vi "_check controller.vi"() -> ()   [LabVIEW 2017]
uses:
  <vilib>/Simulation/Scripting/Companion Diagram/SimConfigNode/SimParams.ctl
  <vilib>/Simulation/Scripting/Companion Diagram/SimConfigNode/_simSolvers.ctl
  <vilib>/Simulation/Implementation/Shared/SIMSCR Execution Mode.ctl
  <vilib>/Simulation/Param Hierarchy/Typedefs/SIMPH Param Control Actions.ctl
  <vilib>/Simulation/Implementation/Shared/NILVSim_ParamChanged.vi
  <vilib>/Simulation/Implementation/Shared/NILVSIM_BeginStep.vi
  <vilib>/Simulation/Implementation/Shared/NILVSim_Manager.vi
  <vilib>/Utility/error.llb/Clear Errors.vi
  <vilib>/Simulation/Implementation/Shared/NILVSim_FinalizeModel.vi
  <vilib>/DAQmx/read.llb/DAQmx Read (Counter DBL 1Chan 1Samp).vi
  <vilib>/DAQmx/read.llb/DAQmx Read (Digital Bool 1Line 1Point).vi
  917b7e52-755f-4d44-bea8-9e7c9beac24e.vi
  a58f9967-76f1-4ebc-ad3d-26e75a3ca160.vi
  <vilib>/DAQmx/write.llb/DAQmx Write (Analog DBL 1Chan 1Samp).vi
  <vilib>/DAQmx/create/channels.llb/DAQmx Create Channel (AO-Voltage-Basic).vi
  <vilib>/DAQmx/create/channels.llb/DAQmx Create Channel (DI-Digital Input).vi
  <vilib>/DAQmx/create/channels.llb/DAQmx Create Channel (CI-Count Edges).vi
  <vilib>/Simulation/Implementation/Shared/SIM Unbundle Sim Info.vi
  <vilib>/Simulation/Implementation/Shared/NILVSim_Initialize.vi
  <vilib>/Simulation/Utility/Implementation/NILVSim Get Time and IsAcceptedStep.vi
  <vilib>/Simulation/Implementation/Shared/SIMSH Read Queue.vi
  <vilib>/Simulation/Implementation/Shared/NILVSim_GetModelError.vi
  <vilib>/Simulation/Implementation/Shared/SIM Bundle Sim Info.vi
  <vilib>/DAQmx/miscellaneous.llb/DAQmx Fill In Error Info.vi
  <vilib>/Simulation/Implementation/XNodeFramework/SimXNode/SimX.xnode
  <vilib>/Simulation/Model Libraries/PID/SIM PID (Parallel).vi
  <vilib>/Simulation/Model Libraries/PID/SIM PID.vi
  <vilib>/Simulation/Scripting/Companion Diagram/SimConfigNode/SimDog.xnode
  <vilib>/Simulation/Model Libraries/PID/SIM PID (Academic).vi
  <vilib>/Simulation/Implementation/Shared/NI_SIM_Implementation.lvlib
panel:
  out "temp height":dbl
  out "Boolean 2":bool
  out "reset":bool
  in  "checking re":bool
  in  "checking enums":T1(ring)
  in  "rectangle":bool
  in  "Boolean":bool
  out "prev index":dbl
  out "Point rectangle is drawing":dbl
  out "Rectangle Y":dbl[](array[numeric])
  out "Rectangle X":dbl[](array[numeric])
  in  "stage rectangle":T2(ring)
  out "Step 2I":bool
  out "Step 2G":bool
  out "Step 2E":bool
  out "stay1":dbl
  out "stay":dbl
  out "calculating error x":dbl
  out "calculating error y":dbl
  in  "origin":bool
  out "Previous Y":dbl
  out "Previous X":dbl
  out "Current Y":dbl
  out "Current X":dbl
  out "previous index":dbl
  out "both/reset enter":bool
  out "reset complete":bool
  out "x circle":bool
  out "y circle":bool
  out "Point circle is drawing":dbl
  out "false":bool
  in  "Radius 2":dbl
  out "No of Points":dbl
  out "Passing Y":dbl
  out "Y array":dbl[](array[numeric])
  out "array Y length 2":dbl
  out "Passing X":dbl
  out "X array":dbl[](array[numeric])
  out "array x Length 2":dbl
  in  "stage circle":T2(ring)
  in  "check instruc":bool
  out "x entered":dbl
  out "y enetred":dbl
  out "greater -1 x":bool
  out "less 1 x":bool
  out "direction selected":dbl
  out "at 2f":bool
  out "Step 2J":bool
  out "Step 2H":bool
  out "Shape drawing steps":enum16{"corner", "1st switch", "reverse"}(ring)
  out "Step 2D":bool
  out "c":bool
  in  "height":dbl
  in  "length":dbl
  in  "part":T3(ring)=enum."a"
  in  "Has encoders been reset?":enum16{"don't reset", "reset"}(ring)
  out "x distance currently being travelled":dbl
  out "y distance currently being travelled":dbl
  out "error calced":dbl
  out "p1 dis 2":dbl
  out "p1 dis":dbl
  out "error y":dbl
  out "calc distance y":dbl
  out "calc distanc x":dbl
  out "error x":dbl
  out "reached y":bool
  out "reached x":bool
  out "Numeric":dbl
  in  "Draw rectangle":bool
  in  "Draw circle":bool
  out "In drawing mode":bool
  in  "Right-Down":bool
  in  "Left-Up":bool
  in  "Left-Down":bool
  in  "Right-Up":bool
  in  "right":bool
  in  "left":bool
  in  "motor 2":dbl(slide)=1.5 scale=-10.0..10.0
  in  "down":bool
  in  "up":bool
  in  "Y Length":dbl=30.0
  in  "X Length":dbl=30.0
  in  "Motor 2 encoder":tag="Dev1/ctr1"
  out "Pulses M2":dbl format="%.2f"
  in  "Motor 1 encoder":tag="Dev1/ctr0"
  out "Pulses M1":dbl format="%.2f"
  out "Right":bool
  out "Bottom":bool
  out "Left":bool
  out "Top":bool
  in  "Switch 4/Line 3":tag="Dev1/port0/line3"
  in  "Switch 3/Line 2":tag="Dev1/port0/line2"
  in  "Switch 2/Line 1":tag="Dev1/port0/line1"
  in  "Switch 1/Line 0":tag="Dev1/port0/line0"
  in  "Motor stop":bool
  in  "Motor 1":tag="Dev1/ao0"
  in  "max Voltage":dbl=10.0
  in  "Min Voltage":dbl=-10.0
  in  "Motor 2":tag="Dev1/ao1"
  in  "motor 1":dbl(slide)=1.5 scale=-10.0..10.0
  in  "stop":bool
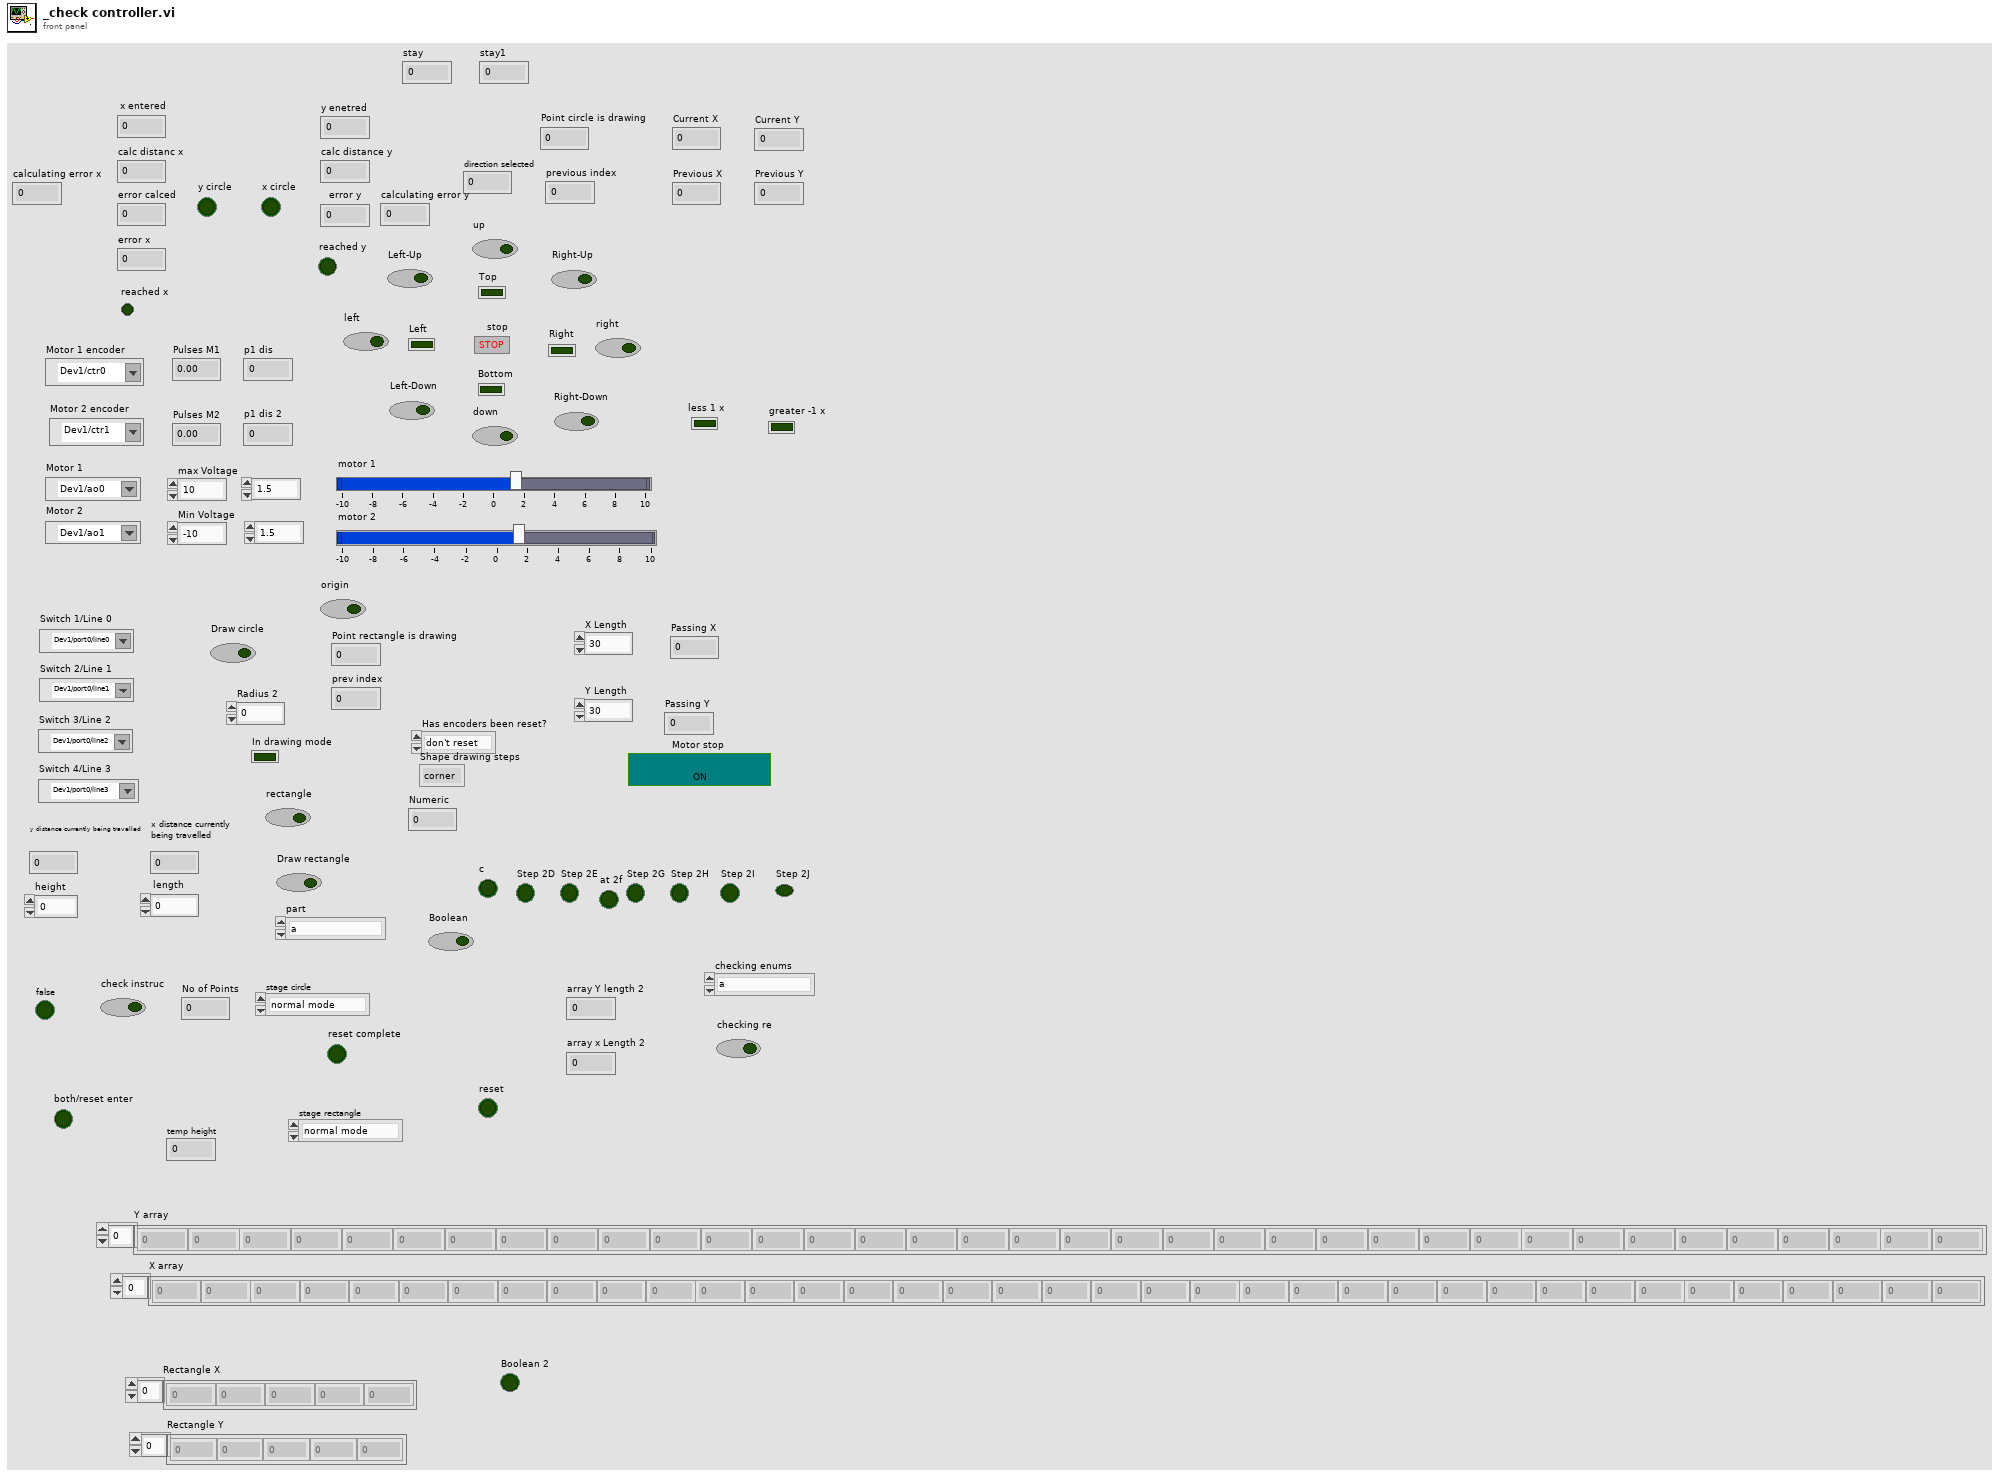
[diagram p1: front panel]
types:
  T1 = enum16{"a", "starting pt", "reset", "going right", "reset before down", "going down", "reset before left", "going left", "reset before up", "going up", "nothing"}
  T2 = enum16{"normal mode", "take to origin", "reset before start", "create points", "draw points", "checking if draw", "reset draw counter"}
  T3 = enum16{"nothing", "j", "i", "h", "g", "f", "e", "d", "c", "b", "a"}
  T4 = enum16{"a", "starting pt", "reset", "going right", "reset before down", "going down", "reset before left", "going left", "reset before up", "going up"}
  T5 = enum16{"Simulate to Completion", "Single Time-Step Simulation (Fixed Step Only)"}
  T6 = typedef "SIMSCR Execution Mode.ctl" = enum16{"Simulate to Completion", "Single Time-Step Simulation (Fixed Step Only)"}
  T7 = typedef "SIMPH Param Control Actions.ctl" = enum16{"get params", "set params"}
  T8 = cluster{"SIMSH Sim Time":dbl, "SIM PID Derivative Gain.vi":cluster{"output":dbl}, "SIM PID Derivative Gain.vi - SIMSH":cluster{"SIMSH Sim Time":dbl, "t 3":dbl, "Select 2":cluster{"s? t:f":dbl}, "Equal?":cluster{"x = y?":bool}, "Or":cluster{"x .or. y?":bool}, "Equal To 0?":cluster{"x = 0?":bool}}, "High Frequency [s] (Tf)":dbl, "Gain":cluster{"output":dbl}, "Summation":cluster{"Result":dbl}, "Integral Gain - series.vi":cluster{"output":dbl}, "Integral Gain - series.vi - SIMSH":cluster{"SIMSH Sim Time":dbl, "Select 2":cluster{"s? t:f":dbl}, "integral in gain?":bool, "Integrator":cluster{"output y(t)":dbl}, "Gain 2":cluster{"output":dbl}, "Select":cluster{"s? t:f":dbl}, "Equal To 0?":cluster{"x = 0?":bool}, "Reciprocal":cluster{"1/x":dbl}}}
  T9 = typedef "SimParams.ctl" = cluster{"Initial Time (s)":dbl, "Final Time (s)":dbl, "Step Size (s)":dbl, "ODE Solver":T10, "Minimum Step Size (s)":dbl, "Maximum Step Size (s)":dbl, "Relative Tolerance":dbl, "Absolute Tolerance":dbl, "Software Timing":bool, "Initial Step Size (s)":dbl, "Automatic Fixed Step Size?":bool, "Automatic Discrete Step Size?":bool, "Discrete Step Size (s)":dbl, "Calculate using Time Step":bool, "Solver Wired?":bool, "Prev.Frm.Expected End":u64, "Prev.Frm.Actual End":u64, "Prev.Frm.Finished Late?":bool, "Prev.Iter.Expected End":u64, "Prev.Iter.Actual End":u64, "Prev.Iter.Finished Late?":bool, "Expected Iteration Start":u64, "Actual Iteration Start":u64, "Expected Frame Start":u64, "Actual Frame Start":u64, "Source Name":string, "Name":string, "Period":i64, "Deadline":i64, "Offset":i64, "Start":i64, "Priority":i32, "Timeout":i32, "Processor":i32, "Mode":enum32{"No Change", "Process missed periods, maintain original phase", "Discard missed periods, maintain original phase", "Process missed periods, ignore original phase", "Discard missed periods, ignore original phase"}, "Wakeup reason":enum32{"Normal", "Aborted", "Asynchronous wakeup", "Timing source error", "Timed loop error", "Timeout"}, "Error":errorcluster, "Source Type":string, "Secondary Source Type":string, "Global End Time":u64, "Global Start Time":u64, "Full Solver Reset":bool, "Execution Mode":T6, "Nan/Inf Check":bool, "Custom Solver Library":string, "Solver Is Variable":bool, "custom solver name":string, "Signal Collection Decimation":u32}
  T10 = typedef "_simSolvers.ctl" = enum16{"Runge-Kutta 1 (Euler)", "Runge-Kutta 2", "Runge-Kutta 3", "Runge-Kutta 4", "Runge-Kutta 23 (variable)", "Runge-Kutta 45 (variable)", "BDF (variable)", "Adams-Moulton (variable)", "Rosenbrock (variable)", "Discrete States Only", "SDIRK 4 (variable)", "Radau 5 (variable)", "Radau 9 (variable)", "Radau 13 (variable)", "Radau [Variable Order] (variable)", "Gear's Method (variable)", "Linearizer", "State Query", "Trim Eval", "Custom Solver"}
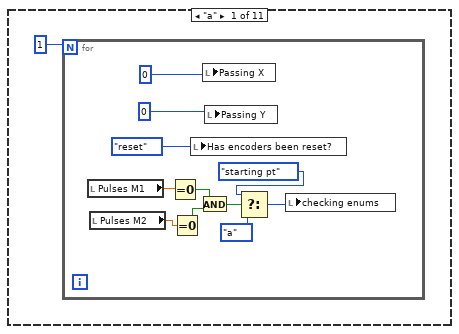
[diagram p3: hidden frame]
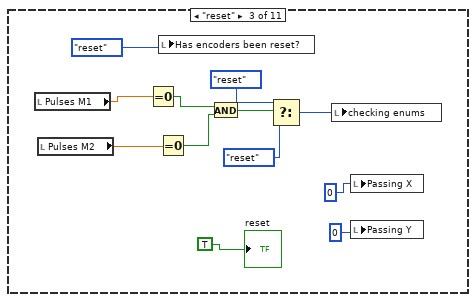
[diagram p4: hidden frame]
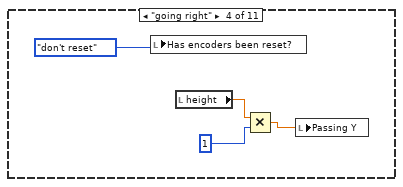
[diagram p5: hidden frame]
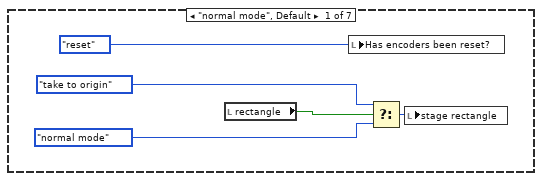
[diagram p14: hidden frame]
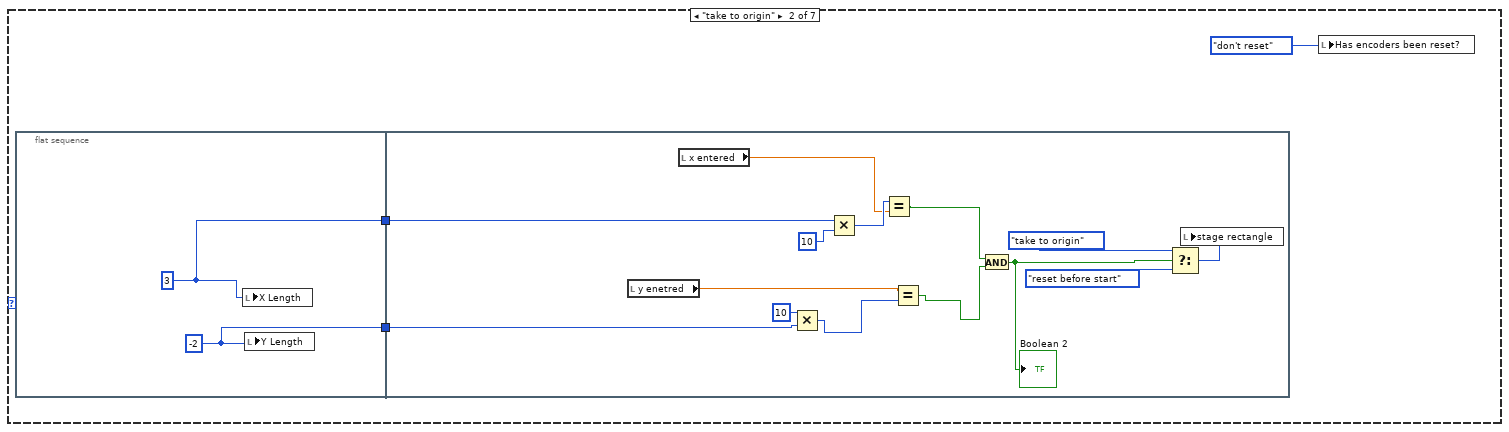
[diagram p15: hidden frame]
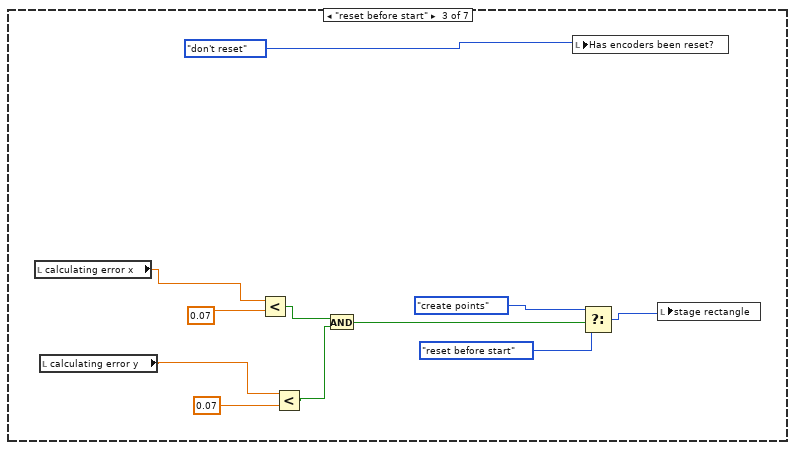
[diagram p16: hidden frame]
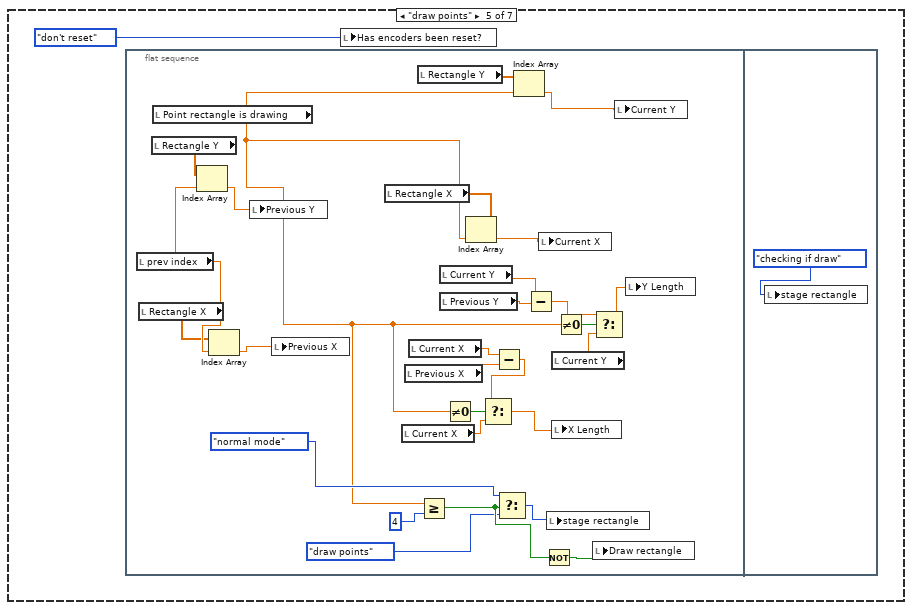
[diagram p17: hidden frame]
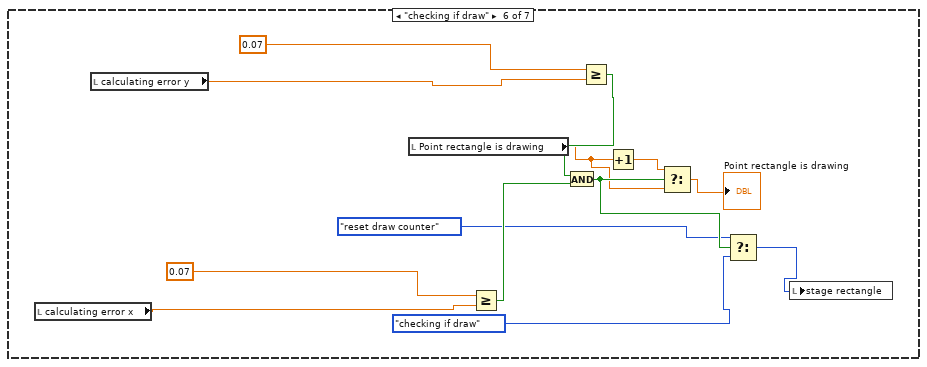
[diagram p18: hidden frame]
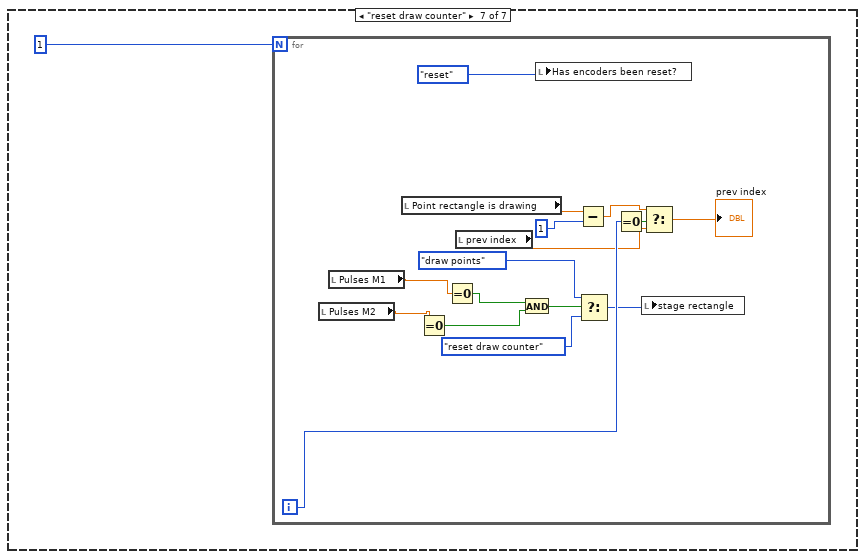
[diagram p19: hidden frame]
diagram:
  n1 = call-poly <vilib>:"DAQmx Create Virtual Channel.vi"("lines"="Switch 1/Line 0") -> ("task out"=w36:refnum<k21>, "error out"=w32:errorcluster)  [unwired: 13 in]
  n2 = call-poly <vilib>:"DAQmx Create Virtual Channel.vi"("lines"="Switch 2/Line 1") -> ("task out"=w35:refnum<k21>, "error out"=w31:errorcluster)  [unwired: 13 in]
  n3 = call-poly <vilib>:"DAQmx Create Virtual Channel.vi"("lines"="Switch 3/Line 2") -> ("task out"=w34:refnum<k21>, "error out"=w30:errorcluster)  [unwired: 13 in]
  n4 = call-poly <vilib>:"DAQmx Create Virtual Channel.vi"("lines"="Switch 4/Line 3") -> ("task out"=w33:refnum<k21>, "error out"=w29:errorcluster)  [unwired: 13 in]
  n5 = call-poly <vilib>:"DAQmx Create Virtual Channel.vi"("maximum value"="max Voltage", "minimum value"="Min Voltage", "physical channels"="Motor 1") -> ("task out"=w46:refnum<k21>, "error out"=w42:errorcluster)  [unwired: 11 in]
  n6 = call <vilib>:"DAQmx Start Task.vi"("task/channels in"=w36, "error in"=w32) -> ("task out"=w28:refnum<k21>, "error out"=w26:errorcluster)  [unwired: 12 in]
  n7 = call <vilib>:"DAQmx Start Task.vi"("task/channels in"=w35, "error in"=w31) -> ("task out"=w24:refnum<k21>, "error out"=w21:errorcluster)  [unwired: 12 in]
  n8 = call-poly <vilib>:"DAQmx Create Virtual Channel.vi"("maximum value"="max Voltage", "minimum value"="Min Voltage", "physical channels"="Motor 2") -> ("task out"=w49:refnum<k21>, "error out"=w41:errorcluster)  [unwired: 11 in]
  n9 = call-poly <vilib>:"DAQmx Create Virtual Channel.vi"("counter"="Motor 1 encoder") -> ("task out"=w7:refnum<k21>, "error out"=w2:errorcluster)  [unwired: 13 in]
  n10 = call-poly <vilib>:"DAQmx Create Virtual Channel.vi"("counter"="Motor 2 encoder") -> ("task out"=w6:refnum<k21>)  [unwired: 13 in, 1 out]
  n11 = call <vilib>:"DAQmx Start Task.vi"("task/channels in"=w34, "error in"=w30) -> ("task out"=w23:refnum<k21>, "error out"=w20:errorcluster)  [unwired: 12 in]
  n12 = call <vilib>:"DAQmx Start Task.vi"("task/channels in"=w33, "error in"=w29) -> ("task out"=w22:refnum<k21>, "error out"=w19:errorcluster)  [unwired: 12 in]
  n13 = call <vilib>:"DAQmx Start Task.vi"("task/channels in"=w7) -> ("task out"=w3:refnum<k21>)  [unwired: 13 in, 1 out]
  n14 = call <vilib>:"DAQmx Start Task.vi"("task/channels in"=w6) -> ("task out"=w1:refnum<k21>)  [unwired: 13 in, 1 out]
  n15 = while {
    tunnel: w49 -> [w242]
    tunnel: [w239] -> w48
    tunnel: w46 -> [w236]
    tunnel: [w235] -> w45
    tunnel: w42 -> [w233]
    tunnel: w41 -> [w232]
    tunnel: w28 -> [w226]
    tunnel: [w225] -> w27
    tunnel: w26 -> [w224]
    tunnel: [w223] -> w25
    tunnel: w24 -> [w222]
    tunnel: w23 -> [w221]
    tunnel: w22 -> [w220]
    tunnel: w21 -> [w219]
    tunnel: w20 -> [w218]
    tunnel: w19 -> [w217]
    tunnel: [w216] -> w18
    tunnel: [w215] -> w17
    tunnel: [w214] -> w16
    tunnel: [w213] -> w15
    tunnel: [w212] -> w14
    tunnel: [w211] -> w13
    tunnel: [w147] -> w10
    tunnel: w3 -> [w149]
    tunnel: w2 -> [w148]
    tunnel: w1 -> [w145]
    stop <- "stop" stop-if-true
    n16 = case shown="True" "check instruc" {
      frame False {
        "false" <- TRUE
      }
      frame True {
        n17 = case shown="\"checking if draw\"" "stage circle" {
          frame "normal mode", Default {
            n18 = local read "check instruc"() -> (w574:bool)
            n19 = local write "Y Length"(0) -> ()
            n20 = local write "X Length"(0) -> ()
            n21 = local write "Has encoders been reset?"(enum16{"don't reset", "reset"}."reset") -> ()
            n22 = Select(t=T2."create points", s=w574, f=T2."normal mode") -> (s? t:f=w575:T2)
            n23 = local write "stage circle"(w575) -> ()
          }
          frame "take to origin" {
            n24 = local write "stage circle"(T2."reset before start") -> ()
            n25 = local write "Has encoders been reset?"(enum16{"don't reset", "reset"}."don't reset") -> ()
          }
          frame "reset before start" {
            n26 = local read "Pulses M1"() -> (w589:dbl)
            n27 = local read "Pulses M2"() -> (w587:dbl)
            n28 = Equal?(x=w589, y=0) -> (x = y?=w584:bool)
            n29 = Equal?(x=w587, y=0) -> (x = y?=w585:bool)
            n30 = local write "Y Length"(0) -> ()
            n31 = local write "X Length"(0) -> ()
            n32 = And(x=w584, y=w585) -> (x .and. y?=w583:bool)
            n33 = local write "Has encoders been reset?"(enum16{"don't reset", "reset"}."reset") -> ()
            n34 = Select(t=T2."create points", s=w583, f=T2."reset before start") -> (s? t:f=w580:T2)
            n35 = local write "stage circle"(w580) -> ()
          }
          frame "create points" {
            n36 = for {
              N: 88 -> [_]
              shift-right: [w609] -> w600
              shift-left: _ -> [_]
              tunnel: [w609] -> w605 mode=indexing
              shift-right: [w608] -> w602
              shift-left: _ -> [_]
              tunnel: [w608] -> w604 mode=indexing
              i -> [w610]
              n37 = Multiply(x=2, y=3.141592653589793) -> (x*y=w613:dbl)
              n38 = Increment(x=w610) -> (x+1=w611:i32)
              n39 = Divide(x=w613, y=88) -> (x/y=w615:dbl)
              n40 = Multiply(x=w615, y=w611) -> (x*y=w612:dbl)
              n41 = Cosine(x=w612) -> (cos(x)=w618:dbl)
              n42 = Sine(x=w612) -> (sin(x)=w619:dbl)
              n43 = Multiply(x=w619, y="Radius 2") -> (x*y=w609:dbl)
              n44 = Multiply(x=w618, y="Radius 2") -> (x*y=w608:dbl)
              "No of Points" <- w610
            }
            "Passing Y" <- w600
            "Y array" <- w605
            "Passing X" <- w602
            "X array" <- w604
            n45 = local read "No of Points"() -> (w599:dbl)
            n46 = Equal?(x=w599, y=87) -> (x = y?=w596:bool)
            n47 = local write "Has encoders been reset?"(enum16{"don't reset", "reset"}."don't reset") -> ()
            n48 = Select(t=T2."draw points", s=w596, f=T2."create points") -> (s? t:f=w606:T2)
            n49 = local write "stage circle"(w606) -> ()
            n50 = Array Size(array=w605) -> (size(s)=→"array Y length 2":i32)
            n51 = Array Size(array=w604) -> (size(s)=→"array x Length 2":i32)
          }
          frame "draw points" {
            n52 = flat-sequence {
              frame #0 {
                n53 = local read "Point circle is drawing"() -> (w648:dbl)
                n54 = local read "previous index"() -> (w640:dbl)
                n55 = local read "Y array"() -> (w641:dbl[])
                n56 = local read "X array"() -> (w642:dbl[])
                n57 = Index Array(array=w641, index=w640) -> (element=→"Previous Y":dbl)
                n58 = Index Array(array=w642, index=w640) -> (element=→"Previous X":dbl)
                n59 = local read "X array"() -> (w643:dbl[])
                n60 = local read "Previous X"() -> (w630:dbl)
                n61 = local read "Current X"() -> (w635:dbl)
                n62 = local read "Y array"() -> (w644:dbl[])
                n63 = local read "Current X"() -> (w633:dbl)
                n64 = Greater Or Equal?(x=w648, y=89) -> (x >= y?=w646:bool)
                n65 = Not Equal To 0?(x=w648) -> (x != 0?=w636:bool)
                n66 = local read "Previous Y"() -> (w631:dbl)
                n67 = local read "Current Y"() -> (w632:dbl)
                n68 = Index Array(array=w643, index=w648) -> (element=→"Current X":dbl)
                n69 = Subtract(x=w633, y=w630) -> (x-y=w628:dbl)
                n70 = Select(t=w628, s=w636, f=w635) -> (s? t:f=w625:dbl)
                n71 = Select(t=T2."normal mode", s=w646, f=T2."draw points") -> (s? t:f=w645:T2)
                n72 = Index Array(array=w644, index=w648) -> (element=→"Current Y":dbl)
                n73 = Subtract(x=w632, y=w631) -> (x-y=w627:dbl)
                n74 = local read "Current Y"() -> (w634:dbl)
                n75 = local write "X Length"(w625) -> ()
                n76 = Not(x=w646) -> (.not. x?=w647:bool)
                n77 = local write "stage circle"(w645) -> ()
                n78 = Not Equal To 0?(x=w648) -> (x != 0?=w637:bool)
                n79 = Select(t=w627, s=w637, f=w634) -> (s? t:f=w626:dbl)
                n80 = local write "Y Length"(w626) -> ()
                n81 = local write "check instruc"(w647) -> ()
              }
              frame #1 {
                n82 = local write "stage circle"(T2."checking if draw") -> ()
              }
            }
            n83 = local write "Has encoders been reset?"(enum16{"don't reset", "reset"}."don't reset") -> ()
          }
          frame "checking if draw" {
            n84 = local read "calculating error x"() -> (w653:dbl)
            n85 = local read "calculating error y"() -> (w651:dbl)
            n86 = local read "Point circle is drawing"() -> (w656:dbl)
            n87 = Greater Or Equal?(x=0.07, y=w653) -> (x >= y?=w659:bool)
            "x circle" <- w659
            n88 = Greater Or Equal?(x=0.07, y=w651) -> (x >= y?=w660:bool)
            "y circle" <- w660
            n89 = And(x=w660, y=w659) -> (x .and. y?=w657:bool)
            "both/reset enter" <- w657
            n90 = Increment(x=w656) -> (x+1=w662:dbl)
            n91 = Select(t=w662, s=w657, f=w656) -> (s? t:f=→"Point circle is drawing":dbl)
            n92 = Select(t=T2."reset draw counter", s=w657, f=T2."checking if draw") -> (s? t:f=w658:T2)
            n93 = local write "stage circle"(w658) -> ()
          }
          frame "reset draw counter" {
            n94 = for {
              N: 1 -> [_]
              i -> [w667]
              n95 = local read "Point circle is drawing"() -> (w672:dbl)
              n96 = local read "Pulses M2"() -> (w677:dbl)
              n97 = local read "Pulses M1"() -> (w678:dbl)
              n98 = Equal To 0?(x=w677) -> (x = 0?=w676:bool)
              n99 = Equal To 0?(x=w678) -> (x = 0?=w674:bool)
              n100 = local read "previous index"() -> (w669:dbl)
              n101 = local write "Has encoders been reset?"(enum16{"don't reset", "reset"}."reset") -> ()
              n102 = And(x=w674, y=w676) -> (x .and. y?=w675:bool)
              n103 = Subtract(x=w672, y=1) -> (x-y=w670:dbl)
              n104 = Select(t=T2."draw points", s=w675, f=T2."reset draw counter") -> (s? t:f=w679:T2)
              n105 = Equal To 0?(x=w667) -> (x = 0?=w666:bool)
              n106 = local write "stage circle"(w679) -> ()
              n107 = Select(t=w670, s=w666, f=w669) -> (s? t:f=→"previous index":dbl)
              "reset complete" <- TRUE
            }
          }
        }
      }
    }
    n108 = case shown="True" "rectangle" {
      frame False {
      }
      frame True {
        n109 = case shown="\"create points\"" "stage rectangle" {
          frame "normal mode", Default {
            n110 = local read "rectangle"() -> (w288:bool)
            n111 = local write "Has encoders been reset?"(enum16{"don't reset", "reset"}."reset") -> ()
            n112 = Select(t=T2."take to origin", s=w288, f=T2."normal mode") -> (s? t:f=w286:T2)
            n113 = local write "stage rectangle"(w286) -> ()
          }
          frame "take to origin" {
            n114 = flat-sequence {
              tunnel: [w295] -> w292
              tunnel: [w294] -> w291
              tunnel: w292 -> [w301]
              tunnel: w291 -> [w300]
              frame #0 {
                w295 = -2
                w294 = 3
                n115 = local write "X Length"(w294) -> ()
                n116 = local write "Y Length"(w295) -> ()
              }
              frame #1 {
                n117 = local read "y enetred"() -> (w304:dbl)
                n118 = local read "x entered"() -> (w298:dbl)
                n119 = Multiply(x=10, y=w301) -> (x*y=w303:i32)
                n120 = Multiply(x=w300, y=10) -> (x*y=w299:i32)
                n121 = Equal?(x=w299, y=w298) -> (x = y?=w297:bool)
                n122 = Equal?(x=w304, y=w303) -> (x = y?=w296:bool)
                n123 = And(x=w297, y=w296) -> (x .and. y?=w309:bool)
                "Boolean 2" <- w309
                n124 = Select(t=T2."take to origin", s=w309, f=T2."reset before start") -> (s? t:f=w308:T2)
                n125 = local write "stage rectangle"(w308) -> ()
              }
            }
            n126 = local write "Has encoders been reset?"(enum16{"don't reset", "reset"}."don't reset") -> ()
          }
          frame "reset before start" {
            n127 = local read "calculating error x"() -> (w312:dbl)
            n128 = local read "calculating error y"() -> (w311:dbl)
            n129 = Less?(x=w312, y=0.07) -> (x < y?=w313:bool)
            n130 = Less?(x=w311, y=0.07) -> (x < y?=w315:bool)
            n131 = And(x=w313, y=w315) -> (x .and. y?=w310:bool)
            n132 = local write "Has encoders been reset?"(enum16{"don't reset", "reset"}."don't reset") -> ()
            n133 = Select(t=T2."create points", s=w310, f=T2."reset before start") -> (s? t:f=w317:T2)
            n134 = local write "stage rectangle"(w317) -> ()
          }
          frame "create points" {
            n135 = local write "Has encoders been reset?"(enum16{"don't reset", "reset"}."reset") -> ()
            n136 = flat-sequence {
              frame #0 {
                n137 = for {
                  N: 1 -> [_]
                  n138 = local read "Rectangle X"() -> (w361:dbl[])
                  n139 = local read "temp height"() -> (w323:dbl)
                  n140 = local read "Rectangle X"() -> (w348:dbl[])
                  n141 = local read "Rectangle X"() -> (w342:dbl[])
                  n142 = local read "Rectangle Y"() -> (w345:dbl[])
                  n143 = local read "Rectangle Y"() -> (w351:dbl[])
                  n144 = local read "length"() -> (w356:dbl)
                  n145 = Insert Into Array(array=w348, index=0, new element=0) -> (→"Rectangle X":dbl[])
                  n146 = Insert Into Array(array=w345, index=0, new element=0) -> (→"Rectangle Y":dbl[])
                  n147 = Insert Into Array(array=w361, index=2, new element=w356) -> (w358:dbl[])
                  n148 = Insert Into Array(array=w351, index=2, new element=w323) -> (w352:dbl[])
                  n149 = Insert Into Array(array=w342, index=4, new element=0) -> (w343:dbl[])
                  n150 = local write "Rectangle X"(w358) -> ()
                  n151 = local write "Rectangle Y"(w352) -> ()
                  n152 = local write "Rectangle X"(w343) -> ()
                  n153 = local read "Rectangle X"() -> (w360:dbl[])
                  n154 = local read "temp height"() -> (w324:dbl)
                  n155 = local read "Rectangle Y"() -> (w349:dbl[])
                  n156 = local read "Rectangle X"() -> (w362:dbl[])
                  n157 = local read "Rectangle Y"() -> (w341:dbl[])
                  n158 = local read "Rectangle Y"() -> (w354:dbl[])
                  n159 = local read "length"() -> (w355:dbl)
                  n160 = Insert Into Array(array=w349, index=1, new element=w324) -> (w350:dbl[])
                  n161 = Insert Into Array(array=w360, index=1, new element=0) -> (w357:dbl[])
                  n162 = Insert Into Array(array=w341, index=4, new element=0) -> (w344:dbl[])
                  n163 = Insert Into Array(array=w354, index=3, new element=0) -> (w353:dbl[])
                  n164 = local write "Rectangle Y"(w350) -> ()
                  n165 = Insert Into Array(array=w362, index=3, new element=w355) -> (w359:dbl[])
                  n166 = local write "Rectangle X"(w357) -> ()
                  n167 = local write "Rectangle Y"(w353) -> ()
                  n168 = local write "Rectangle X"(w359) -> ()
                  n169 = local write "Rectangle Y"(w344) -> ()
                }
              }
              frame #1 {
                n170 = local read "Rectangle X"() -> (w369:dbl[])
                n171 = local read "Rectangle X"() -> (w390:dbl[])
                n172 = local read "Rectangle Y"() -> (w368:dbl[])
                n173 = local read "Rectangle Y"() -> (w389:dbl[])
                n174 = local read "height"() -> (w388:dbl)
                n175 = local read "length"() -> (w384:dbl)
                n176 = Index Array(array=w390, index=2) -> (element=w385:dbl)
                n177 = Index Array(array=w389, index=2) -> (element=w386:dbl)
                n178 = Index Array(array=w369, index=2) -> (element=w374:dbl)
                n179 = Index Array(array=w368, index=2) -> (element=w375:dbl)
                n180 = Multiply(x=w388, y=-1) -> (x*y=w387:dbl)
                n181 = Equal?(x=w385, y=w384) -> (x = y?=w383:bool)
                n182 = Equal?(x=w386, y=w387) -> (x = y?=w382:bool)
                n183 = Equal?(x=w374, y=0) -> (x = y?=w373:bool)
                n184 = Equal?(x=w375, y=0) -> (x = y?=w372:bool)
                n185 = And(x=w383, y=w382) -> (x .and. y?=w365:bool)
                n186 = And(x=w373, y=w372) -> (x .and. y?=w364:bool)
                n187 = And(x=w365, y=w364) -> (x .and. y?=w363:bool)
                n188 = Select(t=T2."draw points", s=w363, f=T2."create points") -> (s? t:f=w381:T2)
                n189 = local write "stage rectangle"(w381) -> ()
              }
            }
          }
          frame "draw points" {
            n190 = flat-sequence {
              frame #0 {
                n191 = local read "prev index"() -> (w400:dbl)
                n192 = local read "Rectangle X"() -> (w398:dbl[])
                n193 = local read "Rectangle Y"() -> (w399:dbl[])
                n194 = local read "Point rectangle is drawing"() -> (w401:dbl)
                n195 = Index Array(array=w399, index=w400) -> (element=w409:dbl)
                n196 = Index Array(array=w398, index=w400) -> (element=w408:dbl)
                n197 = local write "Previous Y"(w409) -> ()
                n198 = local write "Previous X"(w408) -> ()
                n199 = local read "Rectangle X"() -> (w396:dbl[])
                n200 = local read "Current X"() -> (w403:dbl)
                n201 = local read "Previous X"() -> (w407:dbl)
                n202 = local read "Current X"() -> (w404:dbl)
                n203 = local read "Rectangle Y"() -> (w397:dbl[])
                n204 = Greater Or Equal?(x=w401, y=4) -> (x >= y?=w419:bool)
                n205 = local read "Current Y"() -> (w405:dbl)
                n206 = local read "Previous Y"() -> (w406:dbl)
                n207 = Not Equal To 0?(x=w401) -> (x != 0?=w417:bool)
                n208 = Index Array(array=w396, index=w401) -> (element=w411:dbl)
                n209 = Subtract(x=w404, y=w407) -> (x-y=w415:dbl)
                n210 = Select(t=w415, s=w417, f=w403) -> (s? t:f=w393:dbl)
                n211 = Select(t=T2."normal mode", s=w419, f=T2."draw points") -> (s? t:f=w392:T2)
                n212 = Index Array(array=w397, index=w401) -> (element=w410:dbl)
                n213 = Subtract(x=w405, y=w406) -> (x-y=w414:dbl)
                n214 = local write "Current X"(w411) -> ()
                n215 = Not(x=w419) -> (.not. x?=w395:bool)
                n216 = local write "stage rectangle"(w392) -> ()
                n217 = local read "Current Y"() -> (w402:dbl)
                n218 = local write "X Length"(w393) -> ()
                n219 = Not Equal To 0?(x=w401) -> (x != 0?=w418:bool)
                n220 = local write "Draw rectangle"(w395) -> ()
                n221 = Select(t=w414, s=w418, f=w402) -> (s? t:f=w394:dbl)
                n222 = local write "Current Y"(w410) -> ()
                n223 = local write "Y Length"(w394) -> ()
              }
              frame #1 {
                n224 = local write "stage rectangle"(T2."checking if draw") -> ()
              }
            }
            n225 = local write "Has encoders been reset?"(enum16{"don't reset", "reset"}."don't reset") -> ()
          }
          frame "checking if draw" {
            n226 = local read "calculating error x"() -> (w422:dbl)
            n227 = local read "calculating error y"() -> (w421:dbl)
            n228 = local read "Point rectangle is drawing"() -> (w423:dbl)
            n229 = Greater Or Equal?(x=0.07, y=w422) -> (x >= y?=w431:bool)
            n230 = Greater Or Equal?(x=0.07, y=w421) -> (x >= y?=w432:bool)
            n231 = And(x=w432, y=w431) -> (x .and. y?=w430:bool)
            n232 = Increment(x=w423) -> (x+1=w433:dbl)
            n233 = Select(t=w433, s=w430, f=w423) -> (s? t:f=→"Point rectangle is drawing":dbl)
            n234 = Select(t=T2."reset draw counter", s=w430, f=T2."checking if draw") -> (s? t:f=w424:T2)
            n235 = local write "stage rectangle"(w424) -> ()
          }
          frame "reset draw counter" {
            n236 = for {
              N: 1 -> [_]
              i -> [w442]
              n237 = local read "Pulses M2"() -> (w440:dbl)
              n238 = local read "Pulses M1"() -> (w439:dbl)
              n239 = local read "Point rectangle is drawing"() -> (w437:dbl)
              n240 = Equal To 0?(x=w440) -> (x = 0?=w446:bool)
              n241 = Equal To 0?(x=w439) -> (x = 0?=w448:bool)
              n242 = local read "prev index"() -> (w441:dbl)
              n243 = And(x=w448, y=w446) -> (x .and. y?=w447:bool)
              n244 = local write "Has encoders been reset?"(enum16{"don't reset", "reset"}."reset") -> ()
              n245 = Subtract(x=w437, y=1) -> (x-y=w449:dbl)
              n246 = Select(t=T2."draw points", s=w447, f=T2."reset draw counter") -> (s? t:f=w438:T2)
              n247 = Equal To 0?(x=w442) -> (x = 0?=w450:bool)
              n248 = local write "stage rectangle"(w438) -> ()
              n249 = Select(t=w449, s=w450, f=w441) -> (s? t:f=→"prev index":dbl)
            }
          }
        }
      }
    }
    n250 = local read "height"() -> (w51:dbl)
    n251 = Negate(x=w51) -> (-x=w52:dbl)
    n252 = local write "temp height"(w52) -> ()
    n253 = case shown="True" "checking re" {
      frame False {
      }
      frame True {
        n254 = case shown="\"starting pt\"" "checking enums" {
          frame "a" {
            n255 = for {
              N: 1 -> [_]
              n256 = local read "Pulses M1"() -> (w252:dbl)
              n257 = local read "Pulses M2"() -> (w251:dbl)
              n258 = Equal To 0?(x=w252) -> (x = 0?=w250:bool)
              n259 = Equal To 0?(x=w251) -> (x = 0?=w245:bool)
              n260 = local write "Has encoders been reset?"(enum16{"don't reset", "reset"}."reset") -> ()
              n261 = And(x=w250, y=w245) -> (x .and. y?=w249:bool)
              n262 = local write "Passing X"(0) -> ()
              n263 = local write "Passing Y"(0) -> ()
              n264 = Select(t=T4."starting pt", s=w249, f=T4."a") -> (s? t:f=w246:T4)
              n265 = local write "checking enums"(w246) -> ()
            }
          }
          frame "starting pt" {
            n266 = flat-sequence {
              frame #0 {
                n267 = local write "Passing Y"(10) -> ()
                n268 = local write "Passing X"(-6) -> ()
              }
            }
            n269 = local read "calculating error x"() -> (w265:dbl)
            n270 = local read "calculating error y"() -> (w263:dbl)
            n271 = local write "Has encoders been reset?"(enum16{"don't reset", "reset"}."don't reset") -> ()
            n272 = Less?(x=w265, y=0.07) -> (x < y?=w260:bool)
            n273 = Less?(x=w263, y=0.07) -> (x < y?=w261:bool)
            n274 = And(x=w260, y=w261) -> (x .and. y?=w259:bool)
            n275 = Select(t=T4."reset", s=w259, f=T4."starting pt") -> (s? t:f=w256:T4)
            n276 = local write "checking enums"(w256) -> ()
          }
          frame "reset" {
            (unwired) 0
            n277 = local read "Pulses M1"() -> (w279:dbl)
            n278 = local read "Pulses M2"() -> (w278:dbl)
            n279 = Equal To 0?(x=w279) -> (x = 0?=w276:bool)
            n280 = Equal To 0?(x=w278) -> (x = 0?=w277:bool)
            n281 = local write "Has encoders been reset?"(enum16{"don't reset", "reset"}."reset") -> ()
            n282 = And(x=w276, y=w277) -> (x .and. y?=w275:bool)
            n283 = Select(t=T4."reset", s=w275, f=T4."reset") -> (s? t:f=w272:T4)
            n284 = local write "checking enums"(w272) -> ()
            n285 = local write "Passing X"(0) -> ()
            n286 = local write "Passing Y"(0) -> ()
            "reset" <- TRUE
          }
          frame "going right" {
            n287 = local write "Has encoders been reset?"(enum16{"don't reset", "reset"}."don't reset") -> ()
            n288 = local read "height"() -> (w282:dbl)
            n289 = Multiply(x=w282, y=1) -> (x*y=w283:dbl)
            n290 = local write "Passing Y"(w283) -> ()
          }
          frame "reset before down" {
          }
          frame "going down" {
          }
          frame "reset before left" {
          }
          frame "going left" {
          }
          frame "reset before up" {
          }
          frame "going up" {
          }
          frame "nothing" {
          }
        }
      }
    }
    n291 = case shown="True" "Boolean" {
      frame False {
      }
      frame True {
        n292 = case shown="\"d\"" "part" {
          frame "a" {
            n293 = for {
              N: 1 -> [_]
              n294 = local read "Pulses M1"() -> (w459:dbl)
              n295 = local read "Pulses M2"() -> (w458:dbl)
              n296 = Equal To 0?(x=w458) -> (x = 0?=w461:bool)
              n297 = Equal To 0?(x=w459) -> (x = 0?=w460:bool)
              n298 = local write "Has encoders been reset?"(enum16{"don't reset", "reset"}."reset") -> ()
              n299 = And(x=w460, y=w461) -> (x .and. y?=w453:bool)
              n300 = local write "Passing X"(0) -> ()
              n301 = local write "Passing Y"(0) -> ()
              n302 = Select(t=T3."b", s=w453, f=T3."a") -> (s? t:f=w456:T3)
              n303 = local write "part"(w456) -> ()
            }
          }
          frame "b" {
            n304 = local read "calculating error x"() -> (w472:dbl)
            n305 = local read "calculating error y"() -> (w469:dbl)
            n306 = Greater?(x=w472, y=0.07) -> (0:w471:bool)
            n307 = Greater?(x=w469, y=0.07) -> (0:w467:bool)
            n308 = local write "Has encoders been reset?"(enum16{"don't reset", "reset"}."don't reset") -> ()
            n309 = local write "Passing Y"(1) -> ()
            n310 = local write "Passing X"(1) -> ()
            n311 = And(x=w471, y=w467) -> (x .and. y?=w474:bool)
            n312 = Select(t=T3."c", s=w474, f=T3."b") -> (s? t:f=w475:T3)
            n313 = local write "part"(w475) -> ()
          }
          frame "c" {
            n314 = for {
              N: 0 -> [_]
              n315 = local read "Pulses M2"() -> (w488:dbl)
              n316 = local read "Pulses M1"() -> (w487:dbl)
              n317 = Equal To 0?(x=w488) -> (x = 0?=w486:bool)
              n318 = Equal To 0?(x=w487) -> (x = 0?=w485:bool)
              n319 = local write "Has encoders been reset?"(enum16{"don't reset", "reset"}."reset") -> ()
              n320 = And(x=w486, y=w485) -> (x .and. y?=w484:bool)
              n321 = Select(t=T3."d", s=w484, f=T3."c") -> (s? t:f=w481:T3)
              n322 = local write "part"(w481) -> ()
            }
            n323 = local write "Passing Y"(0) -> ()
            n324 = local write "Passing X"(0) -> ()
            "c" <- TRUE
          }
          frame "d" {
            n325 = local read "calculating error y"() -> (w491:dbl)
            n326 = Multiply(x="height", y=-1) -> (x*y=w492:dbl)
            n327 = local write "Has encoders been reset?"(enum16{"don't reset", "reset"}."don't reset") -> ()
            n328 = local write "Passing X"(0) -> ()
            n329 = local write "Passing Y"(w492) -> ()
            n330 = Equal To 0?(x=w491) -> (x = 0?=w490:bool)
            "Step 2D" <- w490
            n331 = Select(t=T3."e", s=w490, f=T3."d") -> (s? t:f=w499:T3)
            n332 = local write "part"(w499) -> ()
          }
          frame "e" {
            n333 = for {
              N: 1 -> [_]
              n334 = local read "Pulses M1"() -> (w506:dbl)
              n335 = local read "Pulses M2"() -> (w505:dbl)
              n336 = Equal To 0?(x=w505) -> (x = 0?=w511:bool)
              n337 = Equal To 0?(x=w506) -> (x = 0?=w512:bool)
              n338 = local write "Has encoders been reset?"(enum16{"don't reset", "reset"}."reset") -> ()
              n339 = And(x=w512, y=w511) -> (x .and. y?=w510:bool)
              n340 = Select(t=T3."f", s=w510, f=T3."e") -> (s? t:f=w504:T3)
              n341 = local write "part"(w504) -> ()
              "Step 2E" <- TRUE
            }
            n342 = local write "Passing X"(0) -> ()
            n343 = local write "Passing Y"(0) -> ()
          }
          frame "f" {
            n344 = local read "calculating error x"() -> (w514:dbl)
            n345 = Equal To 0?(x=w514) -> (x = 0?=w513:bool)
            "at 2f" <- w513
            n346 = local write "Passing Y"(0) -> ()
            n347 = local write "Passing X"("length") -> ()
            n348 = local write "Has encoders been reset?"(enum16{"don't reset", "reset"}."don't reset") -> ()
            n349 = Select(t=T3."g", s=w513, f=T3."f") -> (s? t:f=w518:T3)
            n350 = local write "part"(w518) -> ()
          }
          frame "g" {
            n351 = for {
              N: 1 -> [_]
              n352 = local read "Pulses M1"() -> (w526:dbl)
              n353 = local read "Pulses M2"() -> (w525:dbl)
              n354 = Equal To 0?(x=w526) -> (x = 0?=w533:bool)
              n355 = Equal To 0?(x=w525) -> (x = 0?=w532:bool)
              n356 = local write "Has encoders been reset?"(enum16{"don't reset", "reset"}."reset") -> ()
              n357 = And(x=w533, y=w532) -> (x .and. y?=w531:bool)
              n358 = Select(t=T3."h", s=w531, f=T3."g") -> (s? t:f=w528:T3)
              n359 = local write "part"(w528) -> ()
            }
            n360 = local write "Passing X"(0) -> ()
            n361 = local write "Passing Y"(0) -> ()
            "Step 2G" <- TRUE
          }
          frame "h" {
            n362 = local read "height"() -> (w536:dbl)
            n363 = local read "calculating error y"() -> (w534:dbl)
            n364 = local write "Passing X"(0) -> ()
            n365 = local write "Passing Y"(w536) -> ()
            n366 = local write "Has encoders been reset?"(enum16{"don't reset", "reset"}."don't reset") -> ()
            n367 = Equal To 0?(x=w534) -> (x = 0?=w535:bool)
            n368 = Select(t=T3."i", s=w535, f=T3."h") -> (s? t:f=w539:T3)
            n369 = local write "part"(w539) -> ()
            "Step 2H" <- TRUE
          }
          frame "i" {
            n370 = for {
              N: 1 -> [_]
              n371 = local read "Pulses M1"() -> (w549:dbl)
              n372 = local read "Pulses M2"() -> (w548:dbl)
              n373 = Equal To 0?(x=w548) -> (x = 0?=w554:bool)
              n374 = Equal To 0?(x=w549) -> (x = 0?=w555:bool)
              n375 = And(x=w555, y=w554) -> (x .and. y?=w553:bool)
              n376 = local write "Has encoders been reset?"(enum16{"don't reset", "reset"}."reset") -> ()
              n377 = Select(t=T3."j", s=w553, f=T3."i") -> (s? t:f=w547:T3)
              n378 = local write "part"(w547) -> ()
            }
            n379 = local write "Passing Y"(0) -> ()
            n380 = local write "Passing X"(0) -> ()
            "Step 2I" <- TRUE
          }
          frame "j" {
            n381 = local read "calculating error x"() -> (w560:dbl)
            n382 = local read "length"() -> (w557:dbl)
            n383 = Equal To 0?(x=w560) -> (x = 0?=w559:bool)
            n384 = Multiply(x=w557, y=-1) -> (x*y=w556:dbl)
            n385 = local write "Has encoders been reset?"(enum16{"don't reset", "reset"}."don't reset") -> ()
            n386 = local write "Passing Y"(0) -> ()
            n387 = local write "Passing X"(w556) -> ()
            n388 = Select(t=T3."nothing", s=w559, f=T3."j") -> (s? t:f=w563:T3)
            n389 = local write "part"(w563) -> ()
            "Step 2J" <- TRUE
          }
          frame "nothing" {
            n390 = local write "X Length"(0) -> ()
            n391 = local write "Y Length"(0) -> ()
          }
        }
      }
    }
    n392 = local read "y enetred"() -> (w73:dbl)
    n393 = local read "calc distance y"() -> (w72:dbl)
    n394 = local read "calc distanc x"() -> (w71:dbl)
    n395 = local read "x entered"() -> (w70:dbl)
    n396 = local read "stay"() -> (w67:dbl)
    n397 = local read "stay1"() -> (w66:dbl)
    n398 = formula code="if (Ylength==0)\nYerror=0;\n else  \nif(Ylength<0)\nYerror= Ylength+calculating_y_dis;\nelse\nYerror= Ylength-calculating_y_dis;\n\nif (stay==0)\nYerror=0;"("Ylength"=w73, "calculating_y_dis"=w72, "stay"=w67) -> ("Yerror"=→"error y":dbl)
    n399 = formula code="if (desired_xlength==0)\nXerror=0;\nelse\nif(desired_xlength>0)\nXerror=desired_xlength-actual_xLength;\nelse\nXerror=desired_xlength+actual_xLength;\n\nif (stay1==0)\nXerror=0;"("desired_xlength"=w70, "actual_xLength"=w71, "stay1"=w66) -> ("Xerror"=→"error x":dbl)
    n400 = local read "error y"() -> (w119:dbl)
    n401 = local read "error y"() -> (w118:dbl)
    n402 = local read "error x"() -> (w120:dbl)
    n403 = local read "error y"() -> (w134:dbl)
    n404 = local read "error y"() -> (w131:dbl)
    n405 = local read "error x"() -> (w127:dbl)
    n406 = local read "error x"() -> (w126:dbl)
    n407 = local read "error y"() -> (w135:dbl)
    n408 = local read "error x"() -> (w136:dbl)
    n409 = Less Than 0?(x=w119) -> (x < 0?=w117:bool)
    n410 = Less Than 0?(x=w120) -> (x < 0?=w116:bool)
    n411 = Greater Than 0?(x=w118) -> (x > 0?=w115:bool)
    n412 = Less Than 0?(x=w131) -> (x < 0?=w129:bool)
    n413 = Equal To 0?(x=w136) -> (x = 0?=w130:bool)
    n414 = Greater Than 0?(x=w134) -> (x > 0?=w133:bool)
    n415 = local read "error y"() -> (w112:dbl)
    n416 = local read "error x"() -> (w111:dbl)
    n417 = Greater Than 0?(x=w127) -> (x > 0?=w125:bool)
    n418 = Equal To 0?(x=w135) -> (x = 0?=w124:bool)
    n419 = Less Than 0?(x=w126) -> (x < 0?=w123:bool)
    n420 = And(x=w117, y=w116) -> (x .and. y?=w113:bool)
    n421 = And(x=w116, y=w115) -> (x .and. y?=w114:bool)
    n422 = And(x=w133, y=w130) -> (x .and. y?=w132:bool)
    n423 = And(x=w130, y=w129) -> (x .and. y?=w128:bool)
    n424 = local read "error y"() -> (w107:dbl)
    n425 = And(x=w125, y=w124) -> (x .and. y?=w122:bool)
    n426 = And(x=w124, y=w123) -> (x .and. y?=w121:bool)
    n427 = Greater Than 0?(x=w112) -> (x > 0?=w110:bool)
    n428 = Greater Than 0?(x=w111) -> (x > 0?=w108:bool)
    n429 = Less Than 0?(x=w107) -> (x < 0?=w106:bool)
    n430 = And(x=w110, y=w108) -> (x .and. y?=w109:bool)
    n431 = And(x=w108, y=w106) -> (x .and. y?=w105:bool)
    n432 = Select(t=1, s=w132, f=0) -> (s? t:f=w195:i32)
    n433 = Select(t=10, s=w121, f=0) -> (s? t:f=w193:i32)
    n434 = Select(t=2, s=w128, f=0) -> (s? t:f=w194:i32)
    n435 = Select(t=100, s=w109, f=0) -> (s? t:f=w191:i32)
    n436 = Select(t=200, s=w113, f=0) -> (s? t:f=w190:i32)
    n437 = Select(t=20, s=w122, f=0) -> (s? t:f=w192:i32)
    n438 = Select(t=1000, s=w114, f=0) -> (s? t:f=w189:i32)
    n439 = Select(t=2000, s=w105, f=0) -> (s? t:f=w175:i32)
    n440 = Add(x=w195, y=w194) -> (x+y=w188:i32)
    n441 = Add(x=w193, y=w192) -> (x+y=w187:i32)
    n442 = Add(x=w191, y=w190) -> (x+y=w186:i32)
    n443 = Add(x=w189, y=w175) -> (x+y=w174:i32)
    n444 = Add(x=w188, y=w187) -> (x+y=w185:i32)
    n445 = Add(x=w186, y=w174) -> (x+y=w173:i32)
    n446 = call-poly <vilib>:"DAQmx Read.vi"("task/channels in"=w226, "error in"=w224) -> ("task out"=w225:refnum<k21>, "data"=w157:bool, "error out"=w223:errorcluster)  [unwired: 11 in]
    "Top" <- w157
    n447 = call-poly <vilib>:"DAQmx Read.vi"("task/channels in"=w222, "error in"=w219) -> ("task out"=w216:refnum<k21>, "data"=w166:bool, "error out"=w213:errorcluster)  [unwired: 11 in]
    "Bottom" <- w166
    n448 = call-poly <vilib>:"DAQmx Read.vi"("task/channels in"=w221, "error in"=w218) -> ("task out"=w215:refnum<k21>, "data"=w165:bool, "error out"=w212:errorcluster)  [unwired: 11 in]
    "Right" <- w165
    n449 = call-poly <vilib>:"DAQmx Read.vi"("task/channels in"=w220, "error in"=w217) -> ("task out"=w214:refnum<k21>, "data"=w164:bool, "error out"=w211:errorcluster)  [unwired: 11 in]
    "Left" <- w164
    n450 = Add(x=w185, y=w173) -> (x+y=w104:i32)
    "direction selected" <- w104
    n451 = local read "check instruc"() -> (w79:bool)
    n452 = Multiply(x="Y Length", y=10) -> (x*y=w89:dbl)
    "y enetred" <- w89
    n453 = local read "Pulses M1"() -> (w146:dbl)
    n454 = Boolean To (0,1)(Boolean=w79) -> (0, 1=w78:i16)
    n455 = local read "Pulses M2"() -> (w150:dbl)
    n456 = Divide(x=w146, y=52.56) -> (x/y=→"p1 dis":dbl)
    n457 = feedback #1() -> (w86:dbl)  [unwired: 1 in]
    "calc distance y" <- w86
    n458 = formula code="Yerror=  (abs(Ylength)- abs(calculating_y_dis));\nif (Yerror<0.07)\nstay=0;\nif (stay==0)\nYerror=0;"("Ylength"=w89, "calculating_y_dis"=w86, "stay"=1, "circle"=w78) -> ("Yerror"=w138:dbl, "stay"=→"stay":i32)
    n459 = Divide(x=w150, y=52.56) -> (x/y=→"p1 dis 2":dbl)
    n460 = formula code="X=((PulseM1/52.56)+(PulseM2/52.56))/2.0;\nY=((PulseM1/52.56)+(PulseM2/52.56))/2.0;"("PulseM1"=w146, "PulseM2"=w150) -> ("X"=w53:dbl, "Y"=w54:dbl)
    "calc distanc x" <- w53
    n461 = feedback-in #1(w54) -> ()
    n462 = xnode "PID"("Error"=w138) -> ("Output"=w82:dbl)  [unwired: 2 in, 11 out]
    n463 = Multiply(x="X Length", y=10) -> (x*y=w92:dbl)
    "x entered" <- w92
    n464 = formula code="Xerror=(abs(desired_xlength)-abs(actual_xLength));\n\nif (Xerror<0.07)\nstay1 =0;\nif (stay1==0)\nXerror=0;"("actual_xLength"=w53, "desired_xlength"=w92, "stay1"=1) -> ("Xerror"=w137:dbl, "stay1"=→"stay1":i32)
    "error calced" <- w137
    n465 = case shown="2000" w104 {
      tunnel: "motor 1" -> [w1232 w1235 w1238 w1245 w1249 w1253 w1259 w1265 w1271 w1276 w1283]
      tunnel: "motor 2" -> [w1229 w1237 w1240 w1243 w1248 w1251 w1257 w1263 w1269 w1277 w1282]
      tunnel: [w1228 w1237 w1239 w1242 w1248 w1250 w1256 w1262 w1268 w1274 w1281] -> w90
      tunnel: [w1231 w1234 w1238 w1244 w1249 w1252 w1258 w1264 w1270 w1275 w1280] -> w91
      frame 0, Default {
        n466 = Multiply(x=0, y=w1232) -> (x*y=w1231:dbl)
        n467 = Multiply(x=0, y=w1229) -> (x*y=w1228:dbl)
      }
      frame 1 {
        n468 = Multiply(x=-1, y=w1235) -> (x*y=w1234:dbl)
      }
      frame 2 {
        n469 = Multiply(x=-1.003, y=w1240) -> (x*y=w1239:dbl)
      }
      frame 10 {
        n470 = Multiply(x=-1, y=w1245) -> (x*y=w1244:dbl)
        n471 = Multiply(x=-1.1, y=w1243) -> (x*y=w1242:dbl)
      }
      frame 20 {
      }
      frame 100 {
        n472 = Multiply(x=0, y=w1253) -> (x*y=w1252:dbl)
        n473 = Multiply(x=1, y=w1251) -> (x*y=w1250:dbl)
      }
      frame 200 {
        n474 = Multiply(x=0, y=w1259) -> (x*y=w1258:dbl)
        n475 = Multiply(x=-1, y=w1257) -> (x*y=w1256:dbl)
      }
      frame 1000 {
        n476 = Multiply(x=-1, y=w1265) -> (x*y=w1264:dbl)
        n477 = Multiply(x=0, y=w1263) -> (x*y=w1262:dbl)
      }
      frame 2000 {
        n478 = Multiply(x=1, y=w1271) -> (x*y=w1270:dbl)
        n479 = Multiply(x=0, y=w1269) -> (x*y=w1268:dbl)
      }
      frame 4000 {
        n480 = Multiply(x=-1, y=w1276) -> (x*y=w1275:dbl)
        n481 = Multiply(x=0, y=w1277) -> (x*y=w1274:dbl)
      }
      frame 8000 {
        n482 = Multiply(x=-1, y=w1283) -> (x*y=w1280:dbl)
        n483 = Multiply(x=0, y=w1282) -> (x*y=w1281:dbl)
      }
    }
    n484 = Greater?(x=w82, y=-0.07) -> (0:w77:bool)
    n485 = Less?(x=w82, y=0.07) -> (x < y?=w76:bool)
    n486 = local read "Numeric"() -> (w140:dbl)
    n487 = And(x=w77, y=w76) -> (x .and. y?=w99:bool)
    "reached y" <- w99
    n488 = Multiply(x=0, y=w82) -> (x*y=w103:dbl)
    n489 = Select(t=w103, s=w99, f=w82) -> (s? t:f=→"calculating error y":dbl)
    n490 = Or(x=w166, y=w165) -> (x .or. y?=w209:bool)
    n491 = local read "Draw circle"() -> (w144:bool)
    n492 = And(x=w164, y=w157) -> (x .and. y?=w141:bool)
    n493 = local read "rectangle"() -> (w143:bool)
    n494 = Exclusive Or(1:w157, 2:w164) -> (0:w171:bool)
    n495 = Select(t=1, s=w164, f=0) -> (s? t:f=w156:i32)
    n496 = Select(t=2, s=w157, f=w156) -> (s? t:f=w161:i32)
    n497 = local read "check instruc"() -> (w85:bool)
    n498 = local read "Has encoders been reset?"() -> (w87:enum16{"don't reset", "reset"})
    n499 = xnode "PID 2"("Error"=w137) -> ("Output"=w81:dbl)  [unwired: 2 in, 11 out]
    n500 = Or(x=w144, y=w143) -> (x .or. y?=w84:bool)
    n501 = Select(t=1, s=w171, f=w140) -> (s? t:f=w170:dbl)
    n502 = Select(t=2, s=w141, f=w170) -> (s? t:f=w168:dbl)
    n503 = Or(x=w84, y=w85) -> (x .or. y?=w83:bool)
    n504 = Greater?(x=w81, y=-0.07) -> (0:w95:bool)
    "greater -1 x" <- w95
    n505 = Less?(x=w81, y=0.07) -> (x < y?=w96:bool)
    "less 1 x" <- w96
    n506 = call "Number To Enum.vim"("number"=w161, "enum type"=enum16{"Nothing", "Left", "Top"}."Nothing") -> ("number as enum"=w158:enum16{"Nothing", "Left", "Top"})
    n507 = case shown="True" "origin" {
      selector: "origin" -> [w1205 w1213]
      tunnel: [w1205 w1213] -> w172
      tunnel: w158 -> [_ w1206]
      frame False {
      }
      frame True {
        n508 = local read "Numeric"() -> (w1211:dbl)
        n509 = local read "Shape drawing steps"() -> (w1208:enum16{"corner", "1st switch", "reverse"})
        n510 = Equal?(x=w1211, y=2) -> (x = y?=w1210:bool)
        n511 = Select(t=enum16{"corner", "1st switch", "reverse"}."reverse", s=w1210, f=w1208) -> (s? t:f=w1207:enum16{"corner", "1st switch", "reverse"})
        n512 = case shown="\"reverse\"" w1207 {
          tunnel: w1206 -> [_ w1217 _]
          frame "corner" {
            n513 = local write "Y Length"(50) -> ()
            n514 = local write "Has encoders been reset?"(enum16{"don't reset", "reset"}."don't reset") -> ()
            n515 = local write "X Length"(-50) -> ()
          }
          frame "1st switch" {
            n516 = case shown="\"Nothing\", Default" w1217 {
              frame "Nothing", Default {
                n517 = local write "Y Length"(0) -> ()
                n518 = local write "X Length"(0) -> ()
                n519 = local write "Numeric"(2) -> ()
              }
              frame "Left" {
                n520 = local write "X Length"(0) -> ()
                n521 = local write "Y Length"(50) -> ()
              }
              frame "Top" {
                n522 = local write "X Length"(-50) -> ()
                n523 = local write "Y Length"(0) -> ()
              }
            }
            n524 = local write "Has encoders been reset?"(enum16{"don't reset", "reset"}."don't reset") -> ()
          }
          frame "reverse" {
            n525 = local write "Has encoders been reset?"(enum16{"don't reset", "reset"}."reset") -> ()
            "Numeric" <- 2
          }
        }
      }
    }
    "In drawing mode" <- w172
    n526 = case shown="True" w83 {
      tunnel: w149 -> [w693 w698]
      tunnel: w148 -> [w694 w697]
      tunnel: [w691 w696] -> w147
      frame False {
        n527 = call-poly <vilib>:"DAQmx Read.vi"("task/channels in"=w693, "error in"=w694) -> ("data"=w692:dbl, "error out"=w691:errorcluster)  [unwired: 11 in, 1 out]
        n528 = local write "Pulses M1"(w692) -> ()
      }
      frame True {
        n529 = case shown="\"don't reset\", Default" "Has encoders been reset?" {
          tunnel: w698 -> [w702 w709]
          tunnel: w697 -> [w701 w708]
          tunnel: [w699 w710] -> w696
          frame "don't reset", Default {
            n530 = call-poly <vilib>:"DAQmx Read.vi"("task/channels in"=w702, "error in"=w701) -> ("data"=→"Pulses M1":dbl, "error out"=w699:errorcluster)  [unwired: 11 in, 1 out]
          }
          frame "reset" {
            n531 = call <vilib>:"DAQmx Stop Task.vi"("task/channels in"=w709, "error in"=w708) -> ("task out"=w707:refnum<k21>, "error out"=w706:errorcluster)  [unwired: 12 in]
            n532 = call <vilib>:"DAQmx Start Task.vi"("task/channels in"=w707, "error in"=w706) -> ("task out"=w705:refnum<k21>, "error out"=w704:errorcluster)  [unwired: 12 in]
            n533 = call-poly <vilib>:"DAQmx Read.vi"("task/channels in"=w705, "error in"=w704) -> ("data"=w703:dbl, "error out"=w710:errorcluster)  [unwired: 11 in, 1 out]
            n534 = local write "Pulses M1"(w703) -> ()
          }
        }
      }
    }
    n535 = case shown="True" w83 {
      tunnel: w145 -> [w682 w684]
      tunnel: w87 -> [_ w683]
      frame False {
        n536 = call-poly <vilib>:"DAQmx Read.vi"("task/channels in"=w682) -> ("data"=w681:dbl)  [unwired: 12 in, 2 out]
        n537 = local write "Pulses M2"(w681) -> ()
      }
      frame True {
        n538 = case shown="\"don't reset\", Default" w683 {
          tunnel: w684 -> [w686 w689]
          frame "don't reset", Default {
            n539 = call-poly <vilib>:"DAQmx Read.vi"("task/channels in"=w686) -> ("data"=→"Pulses M2":dbl)  [unwired: 12 in, 2 out]
          }
          frame "reset" {
            n540 = call <vilib>:"DAQmx Stop Task.vi"("task/channels in"=w689) -> ("task out"=w688:refnum<k21>)  [unwired: 13 in, 1 out]
            n541 = call <vilib>:"DAQmx Start Task.vi"("task/channels in"=w688) -> ("task out"=w690:refnum<k21>)  [unwired: 13 in, 1 out]
            n542 = call-poly <vilib>:"DAQmx Read.vi"("task/channels in"=w690) -> ("data"=w687:dbl)  [unwired: 12 in, 2 out]
            n543 = local write "Pulses M2"(w687) -> ()
          }
        }
      }
    }
    n544 = call "Number To Enum.vim"("number"=w168, "enum type"=enum16{"corner", "1st switch", "reverse"}."corner") -> ("number as enum"=→"Shape drawing steps":enum16{"corner", "1st switch", "reverse"})
    n545 = And(x=w95, y=w96) -> (x .and. y?=w98:bool)
    n546 = Multiply(x=0, y=w81) -> (x*y=w101:dbl)
    n547 = feedback-in #2(w98) -> ()
    n548 = feedback #2() -> (w97:bool)  [unwired: 1 in]
    "reached x" <- w97
    n549 = And(x=w99, y=w97) -> (x .and. y?=w155:bool)
    n550 = Or(x=w209, y=w155) -> (x .or. y?=w208:bool)
    n551 = Or(x=w208, y="Motor stop") -> (x .or. y?=w210:bool)
    n552 = Or(x=w210, y="stop") -> (x .or. y?=w230:bool)
    n553 = Select(t=0.0, s=w230, f=w90) -> (s? t:f=w227:dbl)
    n554 = call-poly <vilib>:"DAQmx Write.vi"("task/channels in"=w236, "data"=w227, "error in"=w233) -> ("task out"=w237:refnum<k21>, "error out"=w238:errorcluster)  [unwired: 10 in, 1 out]
    n555 = Select(t=0.0 ("s? t:f"), s=w230, f=w91) -> (s? t:f=w228:dbl)
    n556 = call-poly <vilib>:"DAQmx Write.vi"("task/channels in"=w242, "data"=w228, "error in"=w232) -> ("task out"=w241:refnum<k21>, "error out"=w240:errorcluster)  [unwired: 10 in, 1 out]
    n557 = call <vilib>:"DAQmx Wait Until Done.vi"("task/channels in"=w241, "error in"=w240) -> ("error out"=w239:errorcluster)  [unwired: 12 in, 1 out]
    n558 = call <vilib>:"DAQmx Wait Until Done.vi"("task/channels in"=w237, "error in"=w238) -> ("error out"=w235:errorcluster)  [unwired: 12 in, 1 out]
    n559 = Select(t=w101, s=w97, f=w81) -> (s? t:f=→"calculating error x":dbl)
  }
  n560 = invoke on="motor 1" class="Slide (strict)" method="Reinit To Default"() -> ()  [unwired: 3 in, 3 out]
  n561 = invoke on="Numeric" class="DigNum (strict)" method="Reinit To Default"() -> ()  [unwired: 3 in, 3 out]
  n562 = invoke on="No of Points" class="DigNum (strict)" method="Reinit To Default"() -> ()  [unwired: 3 in, 3 out]
  n563 = invoke on="Shape drawing steps" class="Enum (strict)" method="Reinit To Default"() -> ()  [unwired: 3 in, 3 out]
  n564 = invoke on="part" class="Enum (strict)" method="Reinit To Default"() -> ()  [unwired: 3 in, 3 out]
  n565 = invoke on="stage circle" class="Enum (strict)" method="Reinit To Default"() -> ()  [unwired: 3 in, 3 out]
  n566 = invoke on="array Y length 2" class="DigNum (strict)" method="Reinit To Default"() -> ()  [unwired: 3 in, 3 out]
  n567 = invoke on="c" class="Bool (strict)" method="Reinit To Default"() -> ()  [unwired: 3 in, 3 out]
  n568 = invoke on="at 2f" class="Bool (strict)" method="Reinit To Default"() -> ()  [unwired: 3 in, 3 out]
  n569 = invoke on="reached x" class="Bool (strict)" method="Reinit To Default"() -> ()  [unwired: 3 in, 3 out]
  n570 = invoke on="array x Length 2" class="DigNum (strict)" method="Reinit To Default"() -> ()  [unwired: 3 in, 3 out]
  n571 = invoke on="Step 2D" class="Bool (strict)" method="Reinit To Default"() -> ()  [unwired: 3 in, 3 out]
  n572 = invoke on="Step 2H" class="Bool (strict)" method="Reinit To Default"() -> ()  [unwired: 3 in, 3 out]
  n573 = invoke on="Point circle is drawing" class="DigNum (strict)" method="Reinit To Default"() -> ()  [unwired: 3 in, 3 out]
  n574 = invoke on="reached y" class="Bool (strict)" method="Reinit To Default"() -> ()  [unwired: 3 in, 3 out]
  n575 = invoke on="Step 2E" class="Bool (strict)" method="Reinit To Default"() -> ()  [unwired: 3 in, 3 out]
  n576 = invoke on="Step 2J" class="Bool (strict)" method="Reinit To Default"() -> ()  [unwired: 3 in, 3 out]
  n577 = invoke on="previous index" class="DigNum (strict)" method="Reinit To Default"() -> ()  [unwired: 3 in, 3 out]
  n578 = invoke on="Rectangle X" class="Arr (strict)" method="Reinit To Default"() -> ()  [unwired: 3 in, 3 out]
  n579 = invoke on="Rectangle Y" class="Arr (strict)" method="Reinit To Default"() -> ()  [unwired: 3 in, 3 out]
  n580 = call <vilib>:"Simple Error Handler.vi"("error source (\" \")"="you messed up" ("error source (\" \")"), "error in (no error)"=w48) -> ()  [unwired: 3 in, 5 out]
  n581 = call <vilib>:"Simple Error Handler.vi"("error source (\" \")"="you messed up" ("error source (\" \")"), "error in (no error)"=w45) -> ()  [unwired: 3 in, 5 out]
  n582 = call <vilib>:"DAQmx Clear Task.vi"("task in"=w27, "error in"=w25) -> ()  [unwired: 13 in, 1 out]
  n583 = call <vilib>:"DAQmx Clear Task.vi"("task in"=w17, "error in"=w14) -> ()  [unwired: 13 in, 1 out]
  n584 = call <vilib>:"DAQmx Clear Task.vi"("task in"=w18, "error in"=w15) -> ("error out"=w12:errorcluster)  [unwired: 13 in]
  n585 = call <vilib>:"DAQmx Clear Task.vi"("task in"=w16, "error in"=w13) -> ()  [unwired: 13 in, 1 out]
  n586 = call <vilib>:"Simple Error Handler.vi"("error in (no error)"=w12) -> ()  [unwired: 4 in, 5 out]
  n587 = call <vilib>:"Simple Error Handler.vi"("error source (\" \")"="you messed up" ("error source (\" \")"), "error in (no error)"=w10) -> ()  [unwired: 3 in, 5 out]
